vi "Open Next Numbered File.vi"(0 "Dir Path":path=path "/Users/Shared/Data", 1 "Input File Pattern":string="Test") -> (4 "Stop":bool, 5 "Output File Name":string, 6 "refnum out":refnum<file>, 8 "Error Message":string)   [LabVIEW 2019]
doc: "This VI takes a file name and keeps incrementing a tail until it can open a file that does not already exist. Scott Hannahs, FBNML, Jan 1992"
uses:
  <vilib>/Utility/error.llb/DialogType.ctl
panel:
  out "Error Out":errorcluster
  in  "Error In":errorcluster
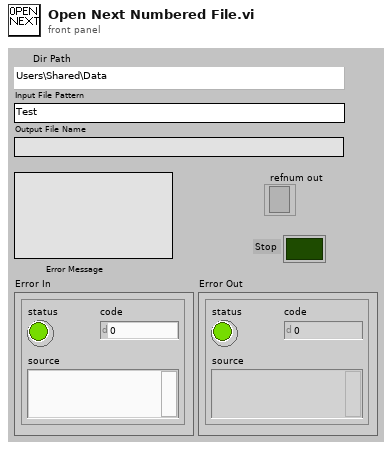
[diagram p1: front panel]
types:
  T1 = typedef "DialogType.ctl" = u16
  T2 = enum16{"open", "replace", "create", "open or create", "replace or create", "replace or create with confirmation"}
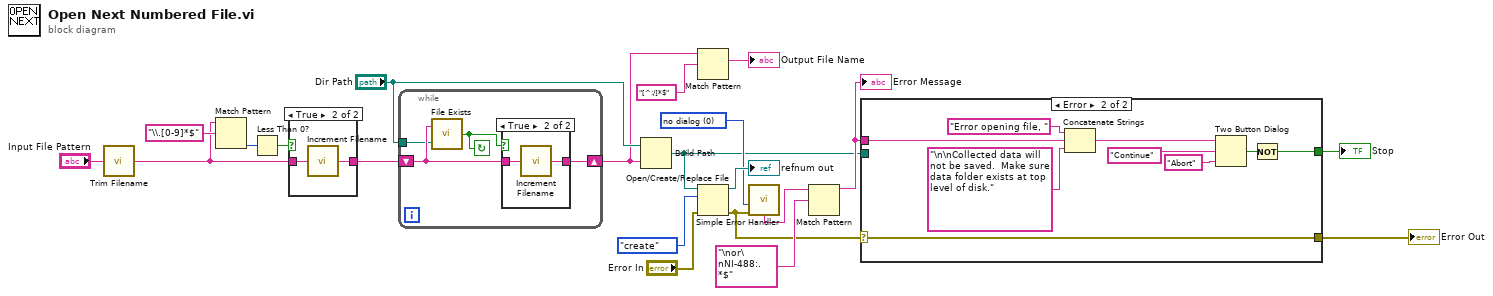
[diagram p0: block diagram]
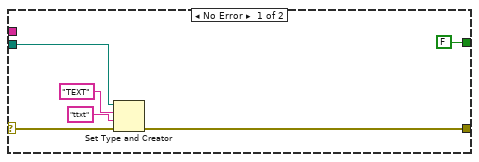
[diagram p3: hidden frame]
diagram:
  w6 = T1 0 items=["no dialog", "OK message", "continue or stop message", "OK message + warnings", "continue/stop + warnings"] ("type of dialog (OK msg:1)")
  n1 = call "Trim Filename.vi"("Input String"="Input File Pattern") -> ("Ouptput String"=w14:string)
  n2 = Match Pattern(string=w14, regular expression="\\.[0-9]*$") -> (offset past match=w21:i32)  [unwired: 1 in, 3 out]
  n3 = Less Than 0?(x=w21) -> (x < 0?=w20:bool)
  n4 = case shown="True" w20 {
    tunnel: [w22 w23] -> w18
    tunnel: w14 -> [w22 w24]
    frame False {
    }
    frame True {
      n5 = call "Increment Filename.vi"("Filename In"=w24) -> ("Filename Out"=w23:string)
    }
  }
  n6 = while {
    tunnel: "Dir Path" -> [w25]
    shift-left: w18 -> [w26]
    shift-right: [w27] -> w7
    stop <- w28 continue-if-true
    n7 = call "File Exists.vi"("Dir Path"=w25, "FILESPEC"=w26) -> (0:w28:bool)
    n8 = case shown="True" w28 {
      tunnel: w26 -> [w29 w30]
      tunnel: [w29 w31] -> w27
      frame False {
      }
      frame True {
        n9 = call "Increment Filename.vi"("Filename In"=w30) -> ("Filename Out"=w31:string)
      }
    }
  }
  n10 = Build Path(base path="Dir Path", name or relative path=w7) -> (appended path=w4:path)
  n11 = Match Pattern(string=w7, regular expression="[^:/]*$") -> (match substring=→"Output File Name":string)  [unwired: 1 in, 3 out]
  n12 = Open/Create/Replace File(file path (use dialog)=w4, error in="Error In", operation (0:open)=T2."create") -> (refnum out=→"refnum out":refnum<file>, error out=w3:errorcluster)  [unwired: 3 in, 1 out]
  n13 = call <vilib>:"Simple Error Handler.vi"("type of dialog (OK msg:1)"=w6, "error in (no error)"=w3) -> ("message"=w12:string)  [unwired: 3 in, 4 out]
  n14 = Match Pattern(string=w12, regular expression="\nor\nNI-488:.*$") -> (before substring=w11:string)  [unwired: 1 in, 3 out]
  "Error Message" <- w11
  n15 = case shown="Error" w3 {
    selector: w3 -> [w33 w38]
    tunnel: w4 -> [w37 _]
    tunnel: w11 -> [_ w42]
    tunnel: [FALSE w43] -> w5
    tunnel: [w32 w38] -> w2
    frame No Error {
      n16 = Set Type and Creator(4:w33, 5:"ttxt", 6:"TEXT", 7:w37) -> (0:w32:errorcluster)  [unwired: 1 out]
    }
    frame Error {
      n17 = Concatenate Strings("Error opening file, ", w42, "\n\nCollected data will not be saved.  Make sure data folder exists at top level of disk.") -> (w39:string)
      n18 = Two Button Dialog(message=w39, 1:"Abort", 2:"Continue") -> (T button?=w45:bool)
      n19 = Not(x=w45) -> (.not. x?=w43:bool)
    }
  }
  "Stop" <- w5
  "Error Out" <- w2
